vi "ABB Efficiency.vi"(11 "auto save":bool) -> ()   [LabVIEW 2017]
uses:
  <vilib>/Analysis/baseanly.llb/Mean (DBL).vi
  ABB global.vi
  <vilib>/Analysis/NI_AALBase.lvlib
panel:
  in  "Slip Entry":dbl[](array[numeric])=[0.0, 0.0, 0.0, 0.0]
  in  "Slip Source":enum16{"Calculated", "Entered"}(ring)
  in  "Specified dTs":cluster{" Stator":string, "Rotor":string}
  in  "Calculated Temperature Rise":cluster{" Stator dT":dbl, "Rotor dT":dbl}
  out "Ambient temp":dbl
  in  "Specified Efficiencies (%)":dbl[](array[numeric])=[0.0, 0.0, 0.0, 0.0]
  in  "Specified  Power Factor":dbl[](array[numeric])=[0.0, 0.0, 0.0, 0.0]
  in  "Temperature Rise Settings":T1
  in  "Frequency (Hz)":dbl
  in  "Remarks":string
  out "Pass/Fail Criteria":string[][](table)
  out "Efficiency Standard":u16(ring) items=["IEC 60034", "NEMA", "IEC 61972"]
  out "Selected Loads (% Rated)":dbl[](array[numeric])
  out "Loads (% Rated)":dbl[](array[numeric])
  out "Efficiency Readings":dbl[][](array[numeric]) format="%#.4f"
  in  "Load selection":bool[](array[boolean])=[FALSE, FALSE, FALSE, FALSE, FALSE]
  out "Stator Resistance/phase":dbl format="%#.6f"
  out "Losses at rated voltage":T2 {"Iron loss" format="%#.2f"; "No-Load Current" format="%#.2f"; "Total No load Power" format="%#.2f"; "Mech Loss" format="%#.3f"}
  out "Rated Data":T3 {"Slip" format="%#.5f"}
  in  "Exit":bool
  # "Efficiency Calculations & Pass/Fail Criteria"
  # "Efficiency"
  # "@"
  # "Calculated slip"
  # "Mechanical Loss  (kW)"
  # "Iron Loss (kW)"
  # "Stator Copper Loss (kW)"
  # "Rotor Copper Loss (kW)"
  # "Stray load loss (kW)"
  # "Total loss (kW)"
  # "Load (kW)"
  # "Efficiency (%)"
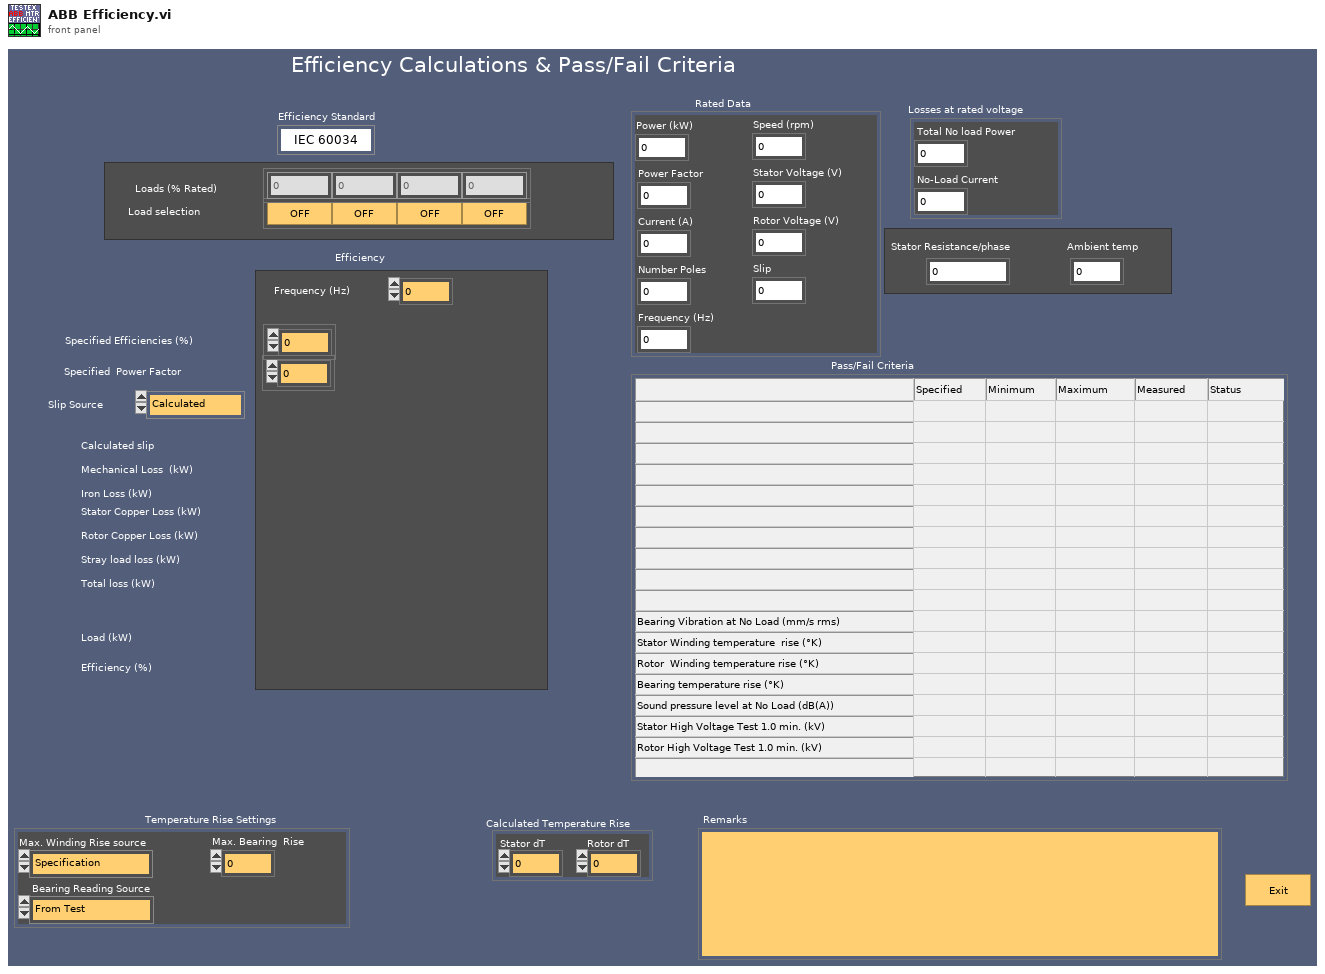
[diagram p1: front panel]
types:
  T1 = cluster{"Max. Winding Rise source":enum16{"Specification", "Enter"}, "Max.Winding Rise":dbl, " Max. Bearing  Rise":dbl, "Bearing Reading Source":enum16{"From Test", "Enter"}, "Bearing reading":dbl}
  T2 = cluster{"Mech Loss":dbl, "Total No load Power":dbl, "No-Load Current":dbl, "Iron loss":dbl}
  T3 = cluster{"Power (kW)":dbl, "Speed (rpm)":dbl, "Power Factor":dbl, "Stator Voltage (V)":dbl, "Current (A)":dbl, "Frequency (Hz)":dbl, "Number Poles":dbl, "Slip":dbl, "Rotor Voltage (V)":dbl}
  T4 = cluster{"Integer":i32, "Dbl":dbl, "String":string, "Boolean":bool}
  T5 = cluster{"Number of Loads":i32, "Loads (%Rated)":dbl[]}
  T6 = cluster{"PCu":dbl, "Pmech":dbl, "PFe":dbl, "Ptot":dbl, "Ambient":dbl, "I1":dbl, "I2":dbl, "I3":dbl, "Wdg Temp":dbl}
  T7 = cluster{"Slip Source":enum16{"Calculated", "Entered"}, "Slip Entry":dbl[]}
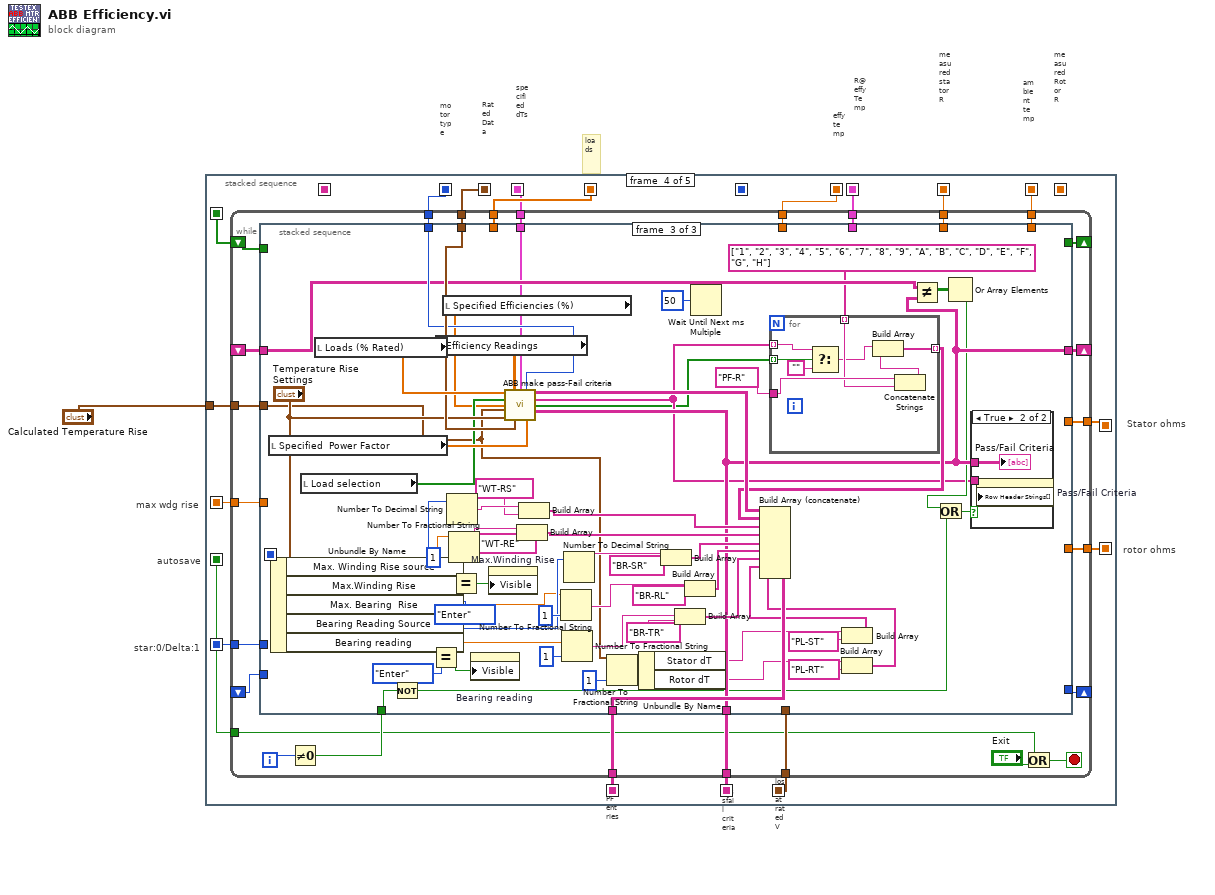
[diagram p0: block diagram]
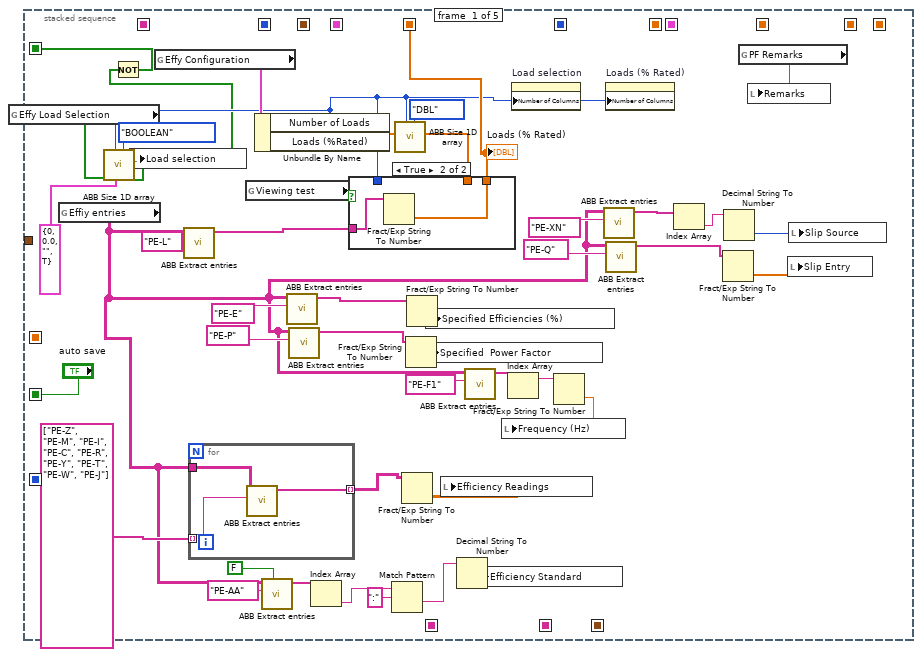
[diagram p2: hidden frame]
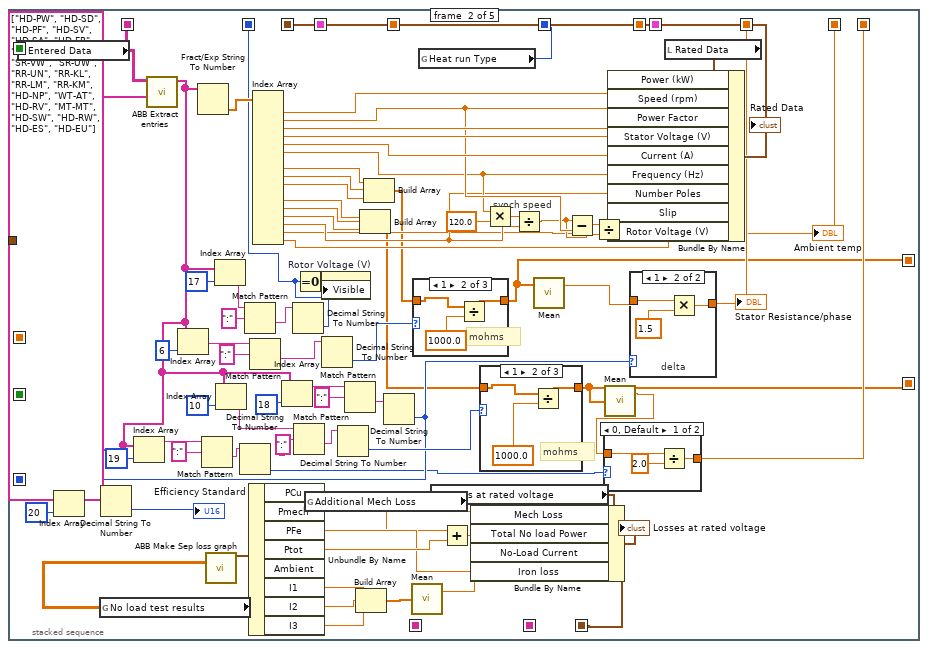
[diagram p4: hidden frame]
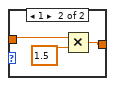
[diagram p5: hidden frame]
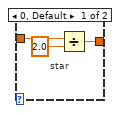
[diagram p6: hidden frame]
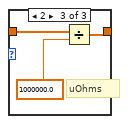
[diagram p8: hidden frame]
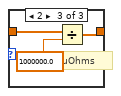
[diagram p10: hidden frame]
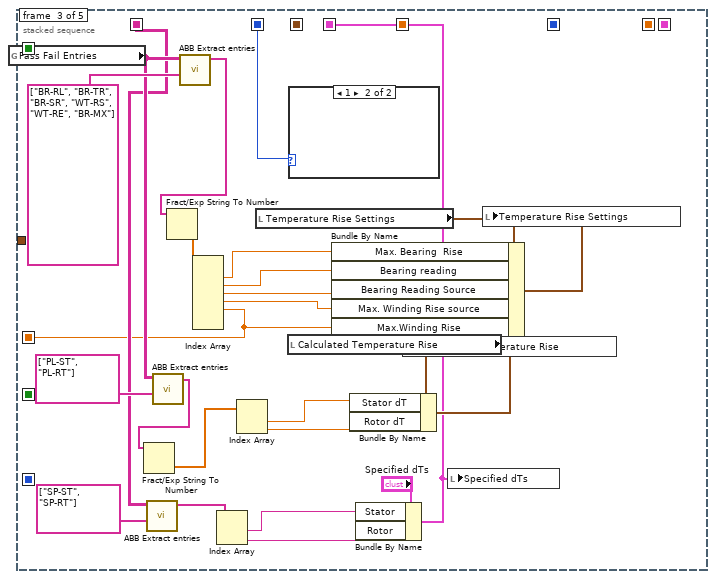
[diagram p11: hidden frame]
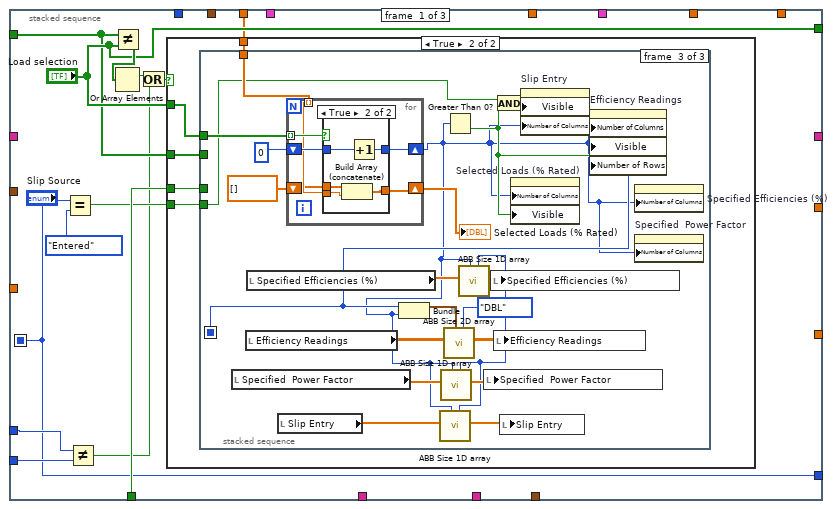
[diagram p13: hidden frame]
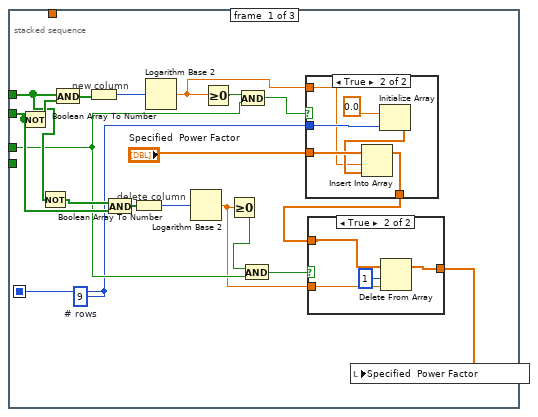
[diagram p15: hidden frame]
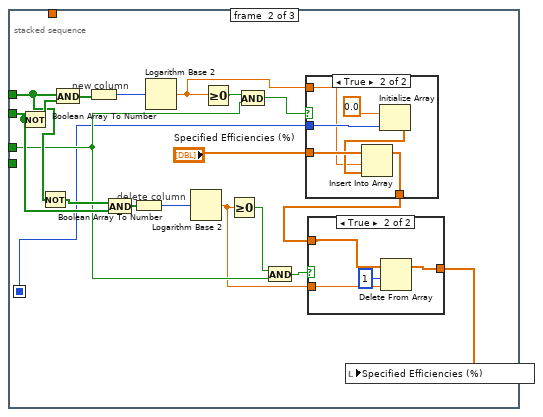
[diagram p18: hidden frame]
diagram:
  # "max wdg rise"
  # "specified dTs"
  # "R@ effy Temp"
  # "rotor ohms"
  # "Stator ohms"
  # "effy temp"
  # "measured Rotor R"
  # "ambient temp"
  # "star:0/Delta:1"
  # "measured stator R"
  # "motor type"
  # "autosave"
  # "PF entries"
  # "passfail criteria"
  # "Rated Data"
  # "losses at rated V"
  # "loads"
  n1 = stacked-sequence {
    seq-local: [w42 _ _ _ _] -> [_ _ _ w199 _]
    seq-local: [w37 _ _ _ _] -> [_ _ _ w198 _]
    seq-local: [_ w110 _ _ _] -> [_ _ _ w197 w432]
    seq-local: [_ w100 _ _ _] -> [_ _ _ w196 _]
    seq-local: [_ _ _ w195 _] -> [_ _ _ _ w438]
    seq-local: [_ _ _ w194 _] -> [_ _ _ _ w437]
    seq-local: [_ w91 _ _ _] -> [_ _ _ _ _]
    seq-local: ["auto save" _ _ _ _] -> [_ _ _ w193 w434]
    seq-local: [_ w81 _ _ _] -> [_ _ w181 w192 _]
    seq-local: [_ w80 _ _ _] -> [_ _ w163 _ _]
    seq-local: [_ w74 _ _ _] -> [_ _ _ w191 _]
    seq-local: [_ w72 _ _ _] -> [_ _ _ w190 _]
    seq-local: [_ w71 _ _ _] -> [_ _ _ w189 _]
    seq-local: [_ w65 _ _ _] -> [_ _ _ _ _]
    seq-local: [_ _ _ w188 _] -> [_ _ _ _ w431]
    seq-local: [_ w60 _ _ _] -> [_ _ _ w186 _]
    seq-local: [_ w59 _ _ _] -> [_ _ _ w185 _]
    seq-local: [_ _ _ w187 _] -> [_ _ _ _ w430]
    seq-local: [_ _ w157 _ _] -> [_ _ _ w184 _]
    seq-local: [_ _ w156 _ _] -> [_ _ _ w183 _]
    tunnel: "Calculated Temperature Rise" -> [_ _ _ w182 _]
    frame #0 {
      n2 = global read "ABB global.vi" "Effy Load Selection"() -> (w14:bool[])
      n3 = global read "ABB global.vi" "Effiy entries"() -> (w4:string[][])
      n4 = global read "ABB global.vi" "Effy Configuration"() -> (w45:T5)
      n5 = call "ABB Extract entries.vi"("Entry ID"="PE-L", "Entry table in"=w4) -> ("Selected Entries"=w39:string[])  [unwired: 9 in]
      n6 = for {
        tunnel: w4 -> [w48]
        tunnel: string[] ["PE-Z", "PE-M", "PE-I", "PE-C", "PE-R", "PE-Y", "PE-T", "PE-W", "PE-J"] -> [w47] mode=indexing
        tunnel: [w46] -> w34 mode=indexing
        n7 = call "ABB Extract entries.vi"("Entry ID"=w47, "Entry table in"=w48) -> ("Selected Entries"=w46:string[])  [unwired: 9 in]
      }
      n8 = global read "ABB global.vi" "Viewing test"() -> (w40:bool)
      n9 = Unbundle By Name(w45) -> ("Number of Loads"=w11:i32, "Loads (%Rated)"=w44:dbl[])
      n10 = call "ABB Size 1D array.vi"("Type"=enum16{"Integer", "DBL", "STRING", "BOOLEAN"}."BOOLEAN", "Default"=T4 {"Integer"=0, "Dbl"=0.0, "String"="", "Boolean"=TRUE}, "Size"=w11, "Boolean Array in"=w14) -> ("Boolean Array out"=w10:bool[])  [unwired: 4 in, 3 out]
      n11 = Not(x=w10) -> (.not. x?=w42:bool[])
      n12 = local write "Load selection"(w10) -> ()
      n13 = call "ABB Extract entries.vi"("Pulldown text"=FALSE, "Entry ID"="PE-AA", "Entry table in"=w4) -> ("Selected Entries"=w30:string[])  [unwired: 8 in]
      n14 = call "ABB Extract entries.vi"("Entry ID"="PE-E", "Entry table in"=w4) -> ("Selected Entries"=w33:string[])  [unwired: 9 in]
      n15 = call "ABB Extract entries.vi"("Entry ID"="PE-P", "Entry table in"=w4) -> ("Selected Entries"=w17:string[])  [unwired: 9 in]
      n16 = Index Array(array=w30) -> (element=w29:string)  [unwired: 1 in]
      n17 = Match Pattern(string=w29, regular expression=":") -> (after substring=w19:string)  [unwired: 1 in, 3 out]
      n18 = call "ABB Size 1D array.vi"("Type"=enum16{"Integer", "DBL", "STRING", "BOOLEAN"}."DBL", "Size"=w11, "DBL Array In"=w44) -> ("DBL Array out"=w38:dbl[])  [unwired: 5 in, 3 out]
      n19 = case shown="True" w40 {
        tunnel: w39 -> [_ w51]
        tunnel: w38 -> [w49 _]
        tunnel: [w49 w50] -> w37
        tunnel: w11 -> [_ _]
        frame False {
        }
        frame True {
          n20 = Fract/Exp String To Number(string=w51) -> (number=w50:dbl[])  [unwired: 3 in, 1 out]
        }
      }
      "Loads (% Rated)" <- w37
      n21 = Fract/Exp String To Number(string=w34) -> (number=w35:dbl[][])  [unwired: 3 in, 1 out]
      n22 = Fract/Exp String To Number(string=w17) -> (number=w16:dbl[])  [unwired: 3 in, 1 out]
      n23 = Fract/Exp String To Number(string=w33) -> (number=w15:dbl[])  [unwired: 3 in, 1 out]
      n24 = local write "Specified  Power Factor"(w16) -> ()
      n25 = local write "Specified Efficiencies (%)"(w15) -> ()
      n26 = local write "Efficiency Readings"(w35) -> ()
      n27 = Decimal String To Number(string=w19) -> (number=w27:i32)  [unwired: 2 in, 1 out]
      n28 = call "ABB Extract entries.vi"("Entry ID"="PE-F1", "Entry table in"=w4) -> ("Selected Entries"=w23:string[])  [unwired: 9 in]
      n29 = local write "Efficiency Standard"(w27) -> ()
      n30 = Index Array(array=w23) -> (element=w22:string)  [unwired: 1 in]
      n31 = property on="Load selection" class="Arr (strict)"("Number of Columns"=w11) -> ()  [unwired: 2 in, 2 out]
      n32 = Fract/Exp String To Number(string=w22) -> (number=w21:dbl)  [unwired: 3 in, 1 out]
      n33 = local write "Frequency (Hz)"(w21) -> ()
      n34 = call "ABB Extract entries.vi"("Entry ID"="PE-XN", "Entry table in"=w4) -> ("Selected Entries"=w5:string[])  [unwired: 9 in]
      n35 = property on="Loads (% Rated)" class="Arr (strict)"("Number of Columns"=w11) -> ()  [unwired: 2 in, 2 out]
      n36 = call "ABB Extract entries.vi"("Entry ID"="PE-Q", "Entry table in"=w4) -> ("Selected Entries"=w8:string[])  [unwired: 9 in]
      n37 = Index Array(array=w5) -> (element=w3:string)  [unwired: 1 in]
      n38 = Fract/Exp String To Number(string=w8) -> (number=w9:dbl[])  [unwired: 3 in, 1 out]
      n39 = Decimal String To Number(string=w3) -> (number=w2:i32)  [unwired: 2 in, 1 out]
      n40 = global read "ABB global.vi" "PF Remarks"() -> (w20:string)
      n41 = local write "Remarks"(w20) -> ()
      n42 = local write "Slip Entry"(w9) -> ()
      n43 = local write "Slip Source"(w2) -> ()
    }
    frame #1 {
      # "synch speed"
      n44 = global read "ABB global.vi" "Entered Data"() -> (w80:string[][])
      n45 = global read "ABB global.vi" "No load test results"() -> (w90:dbl[][])
      n46 = call "ABB Extract entries.vi"("Entry IDs"=string[] ["HD-PW", "HD-SD", "HD-PF", "HD-SV", "HD-SA", "HD-FR", "SR-UN", "SR-UV", "SR-VW", "SR-UW", "RR-UN", "RR-KL", "RR-LM", "RR-KM", "HD-NP", "WT-AT", "HD-RV", "MT-MT", "HD-SW", "HD-RW", "HD-ES", "HD-EU"] ("Array"), "Entry table in"=w80) -> ("Selected Entries"=w57:string[])  [unwired: 9 in]
      n47 = Index Array(array=w57, index=20) -> (element=w56:string)
      n48 = Decimal String To Number(string=w56) -> (number=→"Efficiency Standard":i32)  [unwired: 2 in, 1 out]
      n49 = Index Array(array=w57, index=19) -> (element=w70:string)
      n50 = Index Array(array=w57, index=6) -> (element=w112:string)
      n51 = Fract/Exp String To Number(string=w57) -> (number=w114:dbl[])  [unwired: 3 in, 1 out]
      n52 = Match Pattern(string=w70, regular expression=":") -> (after substring=w66:string)  [unwired: 1 in, 3 out]
      n53 = call "ABB Make Sep loss graph.vi"("Results"=w90) -> ("Rated V Readings"=w124:T6)  [unwired: 8 in, 2 out]
      n54 = Index Array(array=w57, index=17) -> (element=w86:string)
      n55 = Index Array(array=w57, index=10) -> (element=w106:string)
      n56 = Decimal String To Number(string=w66) -> (number=w67:i32)  [unwired: 2 in, 1 out]
      n57 = Match Pattern(string=w86, regular expression=":") -> (after substring=w84:string)  [unwired: 1 in, 3 out]
      n58 = Unbundle By Name(w124) -> ("Pmech"=w52:dbl, "PFe"=w108:dbl, "Ptot"=w123:dbl, "I1"=w122:dbl, "I2"=w121:dbl, "I3"=w120:dbl)  [unwired: 2 out]
      n59 = Match Pattern(string=w112, regular expression=":") -> (after substring=w83:string)  [unwired: 1 in, 3 out]
      n60 = Index Array(array=w114) -> (element #1=w128:dbl, element #2=w99:dbl, element #3=w127:dbl, element #4=w126:dbl, element #5=w125:dbl, element #6=w96:dbl, element #8=w117:dbl, element #9=w116:dbl, element #10=w115:dbl, element #12=w103:dbl, element #13=w102:dbl, element #14=w101:dbl, element #15=w93:dbl, element #16=w71:dbl, element #17=w89:dbl)  [unwired: 17 in, 2 out]
      "Ambient temp" <- w71
      n61 = Index Array(array=w57, index=18) -> (element=w76:string)
      n62 = Decimal String To Number(string=w84) -> (number=w81:i32)  [unwired: 2 in, 1 out]
      n63 = Match Pattern(string=w106, regular expression=":") -> (after substring=w82:string)  [unwired: 1 in, 3 out]
      n64 = Equal To 0?(x=w81) -> (x = 0?=w88:bool)
      n65 = global read "ABB global.vi" "Additional Mech Loss"() -> (w53:dbl)
      n66 = property on="Rotor Voltage (V)" class="DigNum (strict)"("Visible"=w88) -> ()  [unwired: 2 in, 2 out]
      n67 = Decimal String To Number(string=w83) -> (number=w73:i32)  [unwired: 2 in, 1 out]
      n68 = Decimal String To Number(string=w82) -> (number=w104:i32)  [unwired: 2 in, 1 out]
      n69 = Match Pattern(string=w76, regular expression=":") -> (after substring=w78:string)  [unwired: 1 in, 3 out]
      n70 = Build Array(w122, w121, w120) -> (w119:dbl[])
      n71 = Build Array(w103, w102, w101) -> (w62:dbl[])
      n72 = Build Array(w117, w116, w115) -> (w64:dbl[])
      n73 = Decimal String To Number(string=w78) -> (number=w72:i32)  [unwired: 2 in, 1 out]
      n74 = call-poly <vilib>:"Mean.vi"("X"=w119) -> ("mean"=w75:dbl)  [unwired: 1 out]
      n75 = case shown="1" w73 {
        tunnel: w64 -> [w149 w152 w155]
        tunnel: [w149 w150 w153] -> w60
        frame 0, Default {
          # "ohms"
        }
        frame 1 {
          # "mohms"
          n76 = Divide(x=w152, y=1000.0) -> (x/y=w150:dbl[])
        }
        frame 2 {
          # "uOhms"
          n77 = Divide(x=w155, y=1000000.0) -> (x/y=w153:dbl[])
        }
      }
      n78 = global read "ABB global.vi" "Heat run Type"() -> (w91:enum16{"Full Load", "Partial- & No-Load"})
      n79 = local read "Losses at rated voltage"() -> (w129:T2)
      n80 = Add(x=w53, y=w123) -> (x+y=w54:dbl)
      n81 = Bundle By Name(cluster=w129, "Mech Loss"=w52, "Total No load Power"=w54, "No-Load Current"=w75, "Iron loss"=w108) -> (w110:T2)
      "Losses at rated voltage" <- w110
      n82 = case shown="1" w104 {
        tunnel: w62 -> [w142 w145 w148]
        tunnel: [w142 w143 w146] -> w59
        frame 0, Default {
          # "ohms"
        }
        frame 1 {
          # "mohms"
          n83 = Divide(x=w145, y=1000.0) -> (x/y=w143:dbl[])
        }
        frame 2 {
          # "uOhms"
          n84 = Divide(x=w148, y=1000000.0) -> (x/y=w146:dbl[])
        }
      }
      n85 = Multiply(x=w96, y=120.0) -> (x*y=w94:dbl)
      n86 = Divide(x=w94, y=w93) -> (x/y=w92:dbl)
      n87 = call-poly <vilib>:"Mean.vi"("X"=w60) -> ("mean"=w63:dbl)  [unwired: 1 out]
      n88 = Subtract(x=w92, y=w99) -> (x-y=w98:dbl)
      n89 = Divide(x=w98, y=w92) -> (x/y=w97:dbl)
      n90 = call-poly <vilib>:"Mean.vi"("X"=w59) -> ("mean"=w61:dbl)  [unwired: 1 out]
      n91 = case shown="0, Default" w67 {
        tunnel: w61 -> [w131 w133]
        tunnel: [w130 w135] -> w65
        frame 0, Default {
          n92 = Divide(x=w131, y=2.0) -> (x/y=w130:dbl)
        }
        frame 1 {
          n93 = Multiply(x=w133, y=1.5) -> (x*y=w135:dbl)
        }
      }
      n94 = case shown="1" w72 {
        tunnel: w63 -> [w138 w141]
        tunnel: [w136 w140] -> w74
        frame 0, Default {
          # "star"
          n95 = Divide(x=w138, y=2.0) -> (x/y=w136:dbl)
        }
        frame 1 {
          # "delta"
          n96 = Multiply(x=w141, y=1.5) -> (x*y=w140:dbl)
        }
      }
      "Stator Resistance/phase" <- w74
      n97 = local read "Rated Data"() -> (w109:T3)
      n98 = Bundle By Name(cluster=w109, "Power (kW)"=w128, "Speed (rpm)"=w99, "Power Factor"=w127, "Stator Voltage (V)"=w126, "Current (A)"=w125, "Frequency (Hz)"=w96, "Number Poles"=w93, "Slip"=w97, "Rotor Voltage (V)"=w89) -> (w100:T3)
      "Rated Data" <- w100
    }
    frame #2 {
      n99 = global read "ABB global.vi" "Pass Fail Entries"() -> (w169:string[][])
      n100 = call "ABB Extract entries.vi"("Entry IDs"=string[] ["SP-ST", "SP-RT"], "Entry table in"=w163) -> ("Selected Entries"=w161:string[])  [unwired: 9 in]
      n101 = call "ABB Extract entries.vi"("Entry IDs"=string[] ["PL-ST", "PL-RT"], "Entry table in"=w169) -> ("Selected Entries"=w168:string[])  [unwired: 9 in]
      n102 = Fract/Exp String To Number(string=w168) -> (number=w166:dbl[])  [unwired: 3 in, 1 out]
      n103 = call "ABB Extract entries.vi"("Entry IDs"=string[] ["BR-RL", "BR-TR", "BR-SR", "WT-RS", "WT-RE", "BR-MX"], "Entry table in"=w169) -> ("Selected Entries"=w179:string[])  [unwired: 9 in]
      n104 = Fract/Exp String To Number(string=w179) -> (number=w178:dbl[])  [unwired: 3 in, 1 out]
      n105 = Index Array(array=w178) -> (element #1=w175:dbl, element #2=w173:dbl, element #3=w172:dbl, element #4=w174:dbl, element #5=w156:dbl)  [unwired: 7 in, 2 out]
      n106 = Index Array(array=w161) -> (element #1=w159:string, element #2=w158:string)  [unwired: 2 in]
      n107 = Index Array(array=w166) -> (element #1=w165:dbl, element #2=w164:dbl)  [unwired: 2 in]
      n108 = local read "Temperature Rise Settings"() -> (w177:T1)
      n109 = local read "Calculated Temperature Rise"() -> (w171:cluster{" Stator dT":dbl, "Rotor dT":dbl})
      n110 = case shown="1" w181 {
        frame 0, Default {
        }
        frame 1 {
        }
      }
      n111 = Bundle By Name(cluster=w177, "Max. Bearing  Rise"=w175, "Bearing reading"=w173, "Bearing Reading Source"=w172, "Max. Winding Rise source"=w174, "Max.Winding Rise"=w156) -> (w176:T1)
      n112 = Bundle By Name(cluster=w171, "Stator dT"=w165, "Rotor dT"=w164) -> (w170:cluster{" Stator dT":dbl, "Rotor dT":dbl})
      n113 = Bundle By Name(cluster="Specified dTs", "Stator"=w159, "Rotor"=w158) -> (w157:cluster{" Stator":string, "Rotor":string})
      n114 = local write "Calculated Temperature Rise"(w170) -> ()
      n115 = local write "Specified dTs"(w157) -> ()
      n116 = local write "Temperature Rise Settings"(w176) -> ()
    }
    frame #3 {
      n117 = while {
        shift-right: [w224] -> _
        shift-left: w199 -> [w225]
        tunnel: w198 -> [w223]
        tunnel: w197 -> [w220]
        tunnel: w196 -> [w219]
        tunnel: [w218] -> w195
        tunnel: [w217] -> w194
        tunnel: w193 -> [w215]
        tunnel: w192 -> [w214]
        tunnel: w191 -> [w213]
        shift-right: [w211] -> _
        shift-left: _ -> [w212]
        tunnel: w190 -> [w210]
        tunnel: w189 -> [w209]
        tunnel: [w208] -> w188
        tunnel: [w207] -> w187
        tunnel: w186 -> [w206]
        tunnel: w185 -> [w205]
        tunnel: w184 -> [w204]
        shift-right: [w203] -> _
        shift-left: _ -> [w202]
        tunnel: w183 -> [w201]
        tunnel: w182 -> [w200]
        i -> [w222]
        stop <- w216 stop-if-true
        n118 = Not Equal To 0?(x=w222) -> (x != 0?=w221:bool)
        n119 = stacked-sequence {
          seq-local: ["Slip Source" _ _] -> [_ w344 _]
          tunnel: w225 -> [w236 _ _]
          tunnel: ["Load selection" _ _] -> w224
          tunnel: w223 -> [w237 _ _]
          tunnel: w221 -> [w235 _ w379]
          tunnel: w220 -> [_ w356 _]
          tunnel: w219 -> [_ w357 w417]
          tunnel: [_ _ w381] -> w218
          tunnel: [_ _ w412] -> w217
          tunnel: w214 -> [_ _ w414]
          tunnel: w213 -> [_ w355 _]
          tunnel: w212 -> [_ _ w382]
          tunnel: [_ _ w381] -> w211
          tunnel: w210 -> [w231 w352 _]
          tunnel: w209 -> [_ w351 _]
          tunnel: [_ w350 _] -> w208
          tunnel: [_ w349 _] -> w207
          tunnel: w206 -> [_ w348 _]
          tunnel: w205 -> [_ w347 _]
          tunnel: w204 -> [_ _ w361]
          tunnel: ["Slip Source" _ _] -> w203
          tunnel: w202 -> [w232 _ _]
          tunnel: w201 -> [_ _ _]
          tunnel: w200 -> [_ w341 w360]
          frame #0 {
            n120 = Equal?(x="Slip Source", y=enum16{"Calculated", "Entered"}."Entered") -> (x = y?=w233:bool)
            n121 = Not Equal?(x=w231, y=w232) -> (x != y?=w228:bool)
            n122 = Not Equal?(x=w236, y="Load selection") -> (x != y?=w239:bool[])
            n123 = Or Array Elements(Boolean array=w239) -> (logical OR=w229:bool)
            n124 = Or(x=w229, y=w228) -> (x .or. y?=w230:bool)
            n125 = case shown="True" w230 {
              tunnel: "Load selection" -> [_ w243]
              tunnel: w237 -> [_ w244]
              tunnel: w236 -> [_ w242]
              tunnel: w235 -> [_ w241]
              tunnel: w233 -> [_ w240]
              frame False {
              }
              frame True {
                n126 = stacked-sequence {
                  seq-local: [w245 _ _] -> [_ w277 w318]
                  tunnel: w244 -> [_ _ w326]
                  tunnel: w243 -> [w257 w288 w325]
                  tunnel: w242 -> [w255 w286 _]
                  tunnel: w241 -> [w250 w281 _]
                  tunnel: w240 -> [_ _ w311]
                  frame #0 {
                    w245 = 9  # # rows
                    # "delete column"
                    # "new column"
                    n127 = Not(x=w255) -> (.not. x?=w263:bool[])
                    n128 = Not(x=w257) -> (.not. x?=w256:bool[])
                    n129 = And(x=w257, y=w263) -> (x .and. y?=w262:bool[])
                    n130 = Boolean Array To Number(Boolean array=w262) -> (number=w261:u32)
                    n131 = And(x=w256, y=w255) -> (x .and. y?=w253:bool[])
                    n132 = Boolean Array To Number(Boolean array=w253) -> (number=w254:u32)
                    n133 = Logarithm Base 2(1:w261) -> (0:w258:dbl)
                    n134 = Logarithm Base 2(1:w254) -> (0:w248:dbl)
                    n135 = Greater Or Equal To 0?(x=w258) -> (x >= 0?=w260:bool)
                    n136 = Greater Or Equal To 0?(x=w248) -> (x >= 0?=w249:bool)
                    n137 = And(x=w260, y=w250) -> (x .and. y?=w259:bool)
                    n138 = And(x=w249, y=w250) -> (x .and. y?=w251:bool)
                    n139 = case shown="True" w259 {
                      tunnel: "Specified  Power Factor" -> [w269 w275]
                      tunnel: w258 -> [_ w270]
                      tunnel: w245 -> [_ w273]
                      tunnel: [w269 w272] -> w252
                      frame False {
                      }
                      frame True {
                        n140 = Initialize Array(0.0, w273) -> (w271:dbl[])
                        n141 = Insert Into Array(array=w275, index=w270, new element=w271) -> (w272:dbl[])
                      }
                    }
                    n142 = case shown="True" w251 {
                      tunnel: w252 -> [w264 w268]
                      tunnel: w248 -> [_ w265]
                      tunnel: [w264 w267] -> w247
                      frame False {
                      }
                      frame True {
                        n143 = Delete From Array(array=w268, length=1, index=w265) -> (array with subset deleted=w267:dbl[])  [unwired: 1 out]
                      }
                    }
                    n144 = local write "Specified  Power Factor"(w247) -> ()
                  }
                  frame #1 {
                    # "delete column"
                    # "new column"
                    n145 = Not(x=w286) -> (.not. x?=w294:bool[])
                    n146 = Not(x=w288) -> (.not. x?=w287:bool[])
                    n147 = And(x=w288, y=w294) -> (x .and. y?=w293:bool[])
                    n148 = Boolean Array To Number(Boolean array=w293) -> (number=w292:u32)
                    n149 = And(x=w287, y=w286) -> (x .and. y?=w284:bool[])
                    n150 = Boolean Array To Number(Boolean array=w284) -> (number=w285:u32)
                    n151 = Logarithm Base 2(1:w292) -> (0:w289:dbl)
                    n152 = Logarithm Base 2(1:w285) -> (0:w279:dbl)
                    n153 = Greater Or Equal To 0?(x=w289) -> (x >= 0?=w291:bool)
                    n154 = Greater Or Equal To 0?(x=w279) -> (x >= 0?=w280:bool)
                    n155 = And(x=w291, y=w281) -> (x .and. y?=w290:bool)
                    n156 = And(x=w280, y=w281) -> (x .and. y?=w282:bool)
                    n157 = case shown="True" w290 {
                      tunnel: "Specified Efficiencies (%)" -> [w300 w306]
                      tunnel: w289 -> [_ w301]
                      tunnel: w277 -> [_ w304]
                      tunnel: [w300 w303] -> w283
                      frame False {
                      }
                      frame True {
                        n158 = Initialize Array(0.0, w304) -> (w302:dbl[])
                        n159 = Insert Into Array(array=w306, index=w301, new element=w302) -> (w303:dbl[])
                      }
                    }
                    n160 = case shown="True" w282 {
                      tunnel: w283 -> [w295 w299]
                      tunnel: w279 -> [_ w296]
                      tunnel: [w295 w298] -> w278
                      frame False {
                      }
                      frame True {
                        n161 = Delete From Array(array=w299, length=1, index=w296) -> (array with subset deleted=w298:dbl[])  [unwired: 1 out]
                      }
                    }
                    n162 = local write "Specified Efficiencies (%)"(w278) -> ()
                  }
                  frame #2 {
                    w308 = enum16{"Integer", "DBL", "STRING", "BOOLEAN"}."DBL" ("Type")
                    n163 = local read "Specified  Power Factor"() -> (w316:dbl[])
                    n164 = local read "Efficiency Readings"() -> (w319:dbl[][])
                    n165 = local read "Specified Efficiencies (%)"() -> (w315:dbl[])
                    n166 = local read "Slip Entry"() -> (w310:dbl[])
                    n167 = for {
                      tunnel: w326 -> [w329] mode=indexing
                      tunnel: w325 -> [w332] mode=indexing
                      shift-right: [w330] -> w309
                      shift-left: 0 -> [w331]
                      shift-right: [w328] -> w322
                      shift-left: dbl[] [] -> [w327]
                      n168 = case shown="True" w332 {
                        tunnel: w331 -> [w334 w339]
                        tunnel: [w334 w338] -> w330
                        tunnel: w329 -> [_ w336]
                        tunnel: [w333 w335] -> w328
                        tunnel: w327 -> [w333 w337]
                        frame False {
                        }
                        frame True {
                          n169 = Build Array (concatenate)(w337, w336) -> (w335:dbl[])
                          n170 = Increment(x=w339) -> (x+1=w338:i32)
                        }
                      }
                    }
                    "Selected Loads (% Rated)" <- w322
                    n171 = Bundle("# rows"=w318, w309) -> (w321:cluster{"# rows":i32, i32})  [unwired: 1 in]
                    n172 = call "ABB Size 1D array.vi"("Type"=w308, "Size"=w309, "DBL Array In"=w310) -> ("DBL Array out"=w307:dbl[])  [unwired: 5 in, 3 out]
                    n173 = call "ABB Size 1D array.vi"("Type"=w308, "Size"=w309, "DBL Array In"=w316) -> ("DBL Array out"=w317:dbl[])  [unwired: 5 in, 3 out]
                    n174 = call "ABB Size 2D array.vi"("Type"=w308, "Size"=w321, "DBL Array In"=w319) -> ("DBL Array out"=w320:dbl[][])  [unwired: 5 in, 3 out]
                    n175 = Greater Than 0?(x=w309) -> (x > 0?=w313:bool)
                    n176 = call "ABB Size 1D array.vi"("Type"=w308, "Size"=w309, "DBL Array In"=w315) -> ("DBL Array out"=w314:dbl[])  [unwired: 5 in, 3 out]
                    n177 = local write "Specified  Power Factor"(w317) -> ()
                    n178 = local write "Specified Efficiencies (%)"(w314) -> ()
                    n179 = And(x=w311, y=w313) -> (x .and. y?=w312:bool)
                    n180 = local write "Efficiency Readings"(w320) -> ()
                    n181 = local write "Slip Entry"(w307) -> ()
                    n182 = property on="Selected Loads (% Rated)" class="Arr (strict)"("Number of Columns"=w309, "Visible"=w313) -> ()  [unwired: 2 in, 2 out]
                    n183 = property on="Slip Entry" class="Arr (strict)"("Visible"=w312, "Number of Columns"=w309) -> ()  [unwired: 2 in, 2 out]
                    n184 = property on="Efficiency Readings" class="Arr (strict)"("Number of Columns"=w309, "Visible"=w313, "Number of Rows"=w318) -> ()  [unwired: 2 in, 2 out]
                    n185 = property on="Specified Efficiencies (%)" class="Arr (strict)"("Number of Columns"=w309) -> ()  [unwired: 2 in, 2 out]
                    n186 = property on="Specified  Power Factor" class="Arr (strict)"("Number of Columns"=w309) -> ()  [unwired: 2 in, 2 out]
                  }
                }
              }
            }
          }
          frame #1 {
            n187 = Unbundle By Name(w341) -> ("Stator dT"=w340:dbl)
            n188 = local read "Selected Loads (% Rated)"() -> (w358:dbl[])
            n189 = local read "Specified  Power Factor"() -> (w359:dbl[])
            n190 = local read "Efficiency Standard"() -> (w342:u16)
            n191 = local read "Frequency (Hz)"() -> (w354:dbl)
            n192 = Bundle("Slip Source"=w344, "Slip Entry"="Slip Entry") -> (w343:T7)  [unwired: 1 in]
            n193 = Bundle(w348, w347) -> (w346:cluster{dbl[], dbl[]})  [unwired: 1 in]
            n194 = call "ABB Calc efficiency2.vi"("Rated Data"=w357, "max wdg rise"=w340, "Stator wdg"=w352, "Stator  Phase resistance"=w355, "Ambient temp"=w351, "Frequency (Hz)"=w354, "Efficiency Standard"=w342, "Specified  Power Factor"=w359, "Selected Loads (% Rated)"=w358, "Ohms"=w346, "Losses at rated voltage"=w356, "slip entry"=w343) -> ("Efficiency out"=→"Efficiency Readings":dbl[][], "Effy Temp"=w350:dbl, "R at EffyT"=w349:cluster{"Stator":dbl[], "Rotor":dbl[]})  [unwired: 1 in]
          }
          frame #2 {
            n195 = local read "Specified  Power Factor"() -> (w374:dbl[])
            n196 = Unbundle By Name("Temperature Rise Settings") -> ("Max. Winding Rise source"=w406:enum16{"Specification", "Enter"}, "Max.Winding Rise"=w405:dbl, "Max. Bearing  Rise"=w385:dbl, "Bearing Reading Source"=w386:enum16{"From Test", "Enter"}, "Bearing reading"=w384:dbl)
            n197 = local read "Load selection"() -> (w373:bool[])
            n198 = local read "Loads (% Rated)"() -> (w419:dbl[])
            n199 = Not(x=w379) -> (.not. x?=w376:bool)
            n200 = Equal?(x=w386, y=enum16{"From Test", "Enter"}."Enter") -> (x = y?=w407:bool)
            n201 = local read "Efficiency Readings"() -> (w418:dbl[][])
            n202 = local read "Specified Efficiencies (%)"() -> (w371:dbl[])
            n203 = Number To Decimal String(number=w406) -> (decimal integer string=w403:string)  [unwired: 1 in]
            n204 = Number To Fractional String(number=w405, precision (6)=i16 1) -> (F-format string=w402:string)  [unwired: 2 in]
            n205 = Equal?(x=w406, y=enum16{"Specification", "Enter"}."Enter") -> (x = y?=w409:bool)
            n206 = property on="Bearing reading" class="DigNum (strict)"("Visible"=w407) -> ()  [unwired: 2 in, 2 out]
            n207 = property on="Max.Winding Rise" class="DigNum (strict)"("Visible"=w409) -> ()  [unwired: 2 in, 2 out]
            n208 = call "ABB make pass-Fail criteria.vi"("Loads (% Rated)"=w419, "Efficiency Readings"=w418, "spect temp rise"=w361, "motor type"=w414, "Load selection"=w373, "Specified Efficiencies (%)"=w371, "Partial load"=w360, "Temperature Rise Settings"="Temperature Rise Settings", "Rated Data"=w417, "Specified  Power Factor"=w374) -> ("Entries"=w416:string[][], "row headers"=w375:string[], "measurements taken"=w370:bool[], "Pass/Fail Criteria"=w381:string[][])  [unwired: 2 in]
            n209 = Build Array(w402, "WT-RE" ("element")) -> (w398:string[])
            n210 = Build Array(w403, "WT-RS") -> (w399:string[])
            n211 = Number To Fractional String(number=w385, precision (6)=i16 1) -> (F-format string=w394:string)  [unwired: 2 in]
            n212 = Number To Fractional String(number=w384, precision (6)=i16 1) -> (F-format string=w393:string)  [unwired: 2 in]
            n213 = Number To Decimal String(number=w386) -> (decimal integer string=w397:string)  [unwired: 1 in]
            n214 = Number To Fractional String(number=w360, precision (6)=i16 1) -> (F-format string=w369:cluster{" Stator dT":string, "Rotor dT":string})  [unwired: 2 in]
            n215 = Unbundle By Name(w369) -> ("Stator dT"=w366:string, "Rotor dT"=w365:string)
            n216 = Build Array(w397, "BR-SR") -> (w389:string[])
            n217 = Build Array(w393, "BR-TR" ("element")) -> (w387:string[])
            n218 = Build Array(w394, "BR-RL" ("element")) -> (w388:string[])
            n219 = Wait Until Next ms Multiple(millisecond multiple=u32 50) -> ()  [unwired: 1 out]
            n220 = for {
              tunnel: w375 -> [w424] mode=indexing
              tunnel: "PF-R" -> [w429]
              tunnel: [w427] -> w411 mode=indexing
              tunnel: string[] ["1", "2", "3", "4", "5", "6", "7", "8", "9", "A", "B", "C", "D", "E", "F", "G", "H"] -> [w426] mode=indexing
              tunnel: w370 -> [w425] mode=indexing
              n221 = Select(t=w424, s=w425, f="") -> (s? t:f=w422:string)
              n222 = Concatenate Strings(w429, w426) -> (w428:string)
              n223 = Build Array(w422, w428) -> (w427:string[])
            }
            n224 = Build Array(w366, "PL-ST" ("element")) -> (w363:string[])
            n225 = Build Array(w365, "PL-RT" ("element")) -> (w362:string[])
            n226 = Build Array (concatenate)(w416, w411, w399, w398, w389, w388, w387, w363, w362) -> (w412:string[][])
            n227 = Not Equal?(x=w382, y=w381) -> (x != y?=w380:bool[][])
            n228 = Or Array Elements(Boolean array=w380) -> (logical OR=w377:bool)
            n229 = Or(x=w377, y=w376) -> (x .or. y?=w378:bool)
            n230 = case shown="True" w378 {
              tunnel: w381 -> [_ w421]
              tunnel: w375 -> [_ w420]
              frame False {
              }
              frame True {
                n231 = property on="Pass/Fail Criteria" class="Tbl (strict)"("Row Header Strings[]"=w420) -> ()  [unwired: 2 in, 2 out]
                "Pass/Fail Criteria" <- w421
              }
            }
          }
        }
        n232 = Or(x=w215, y="Exit") -> (x .or. y?=w216:bool)
      }
    }
    frame #4 {
      # "No Load Readings\n 0 : I1\n 1 : I2\n 2 : I3\n 3 : Iav\n 4 : V1\n 5 : V2\n 6 : V3\n 7 : Vav\n 8 : Ptot\n 9 : Pf\n10 : Pcu\n11 : Pmech\n12 : Pfe\n13 : Pnold"
      n233 = global read "ABB global.vi" "Viewing test"() -> (w435:bool)
      n234 = Not(x=w434) -> (.not. x?=w433:bool)
      n235 = And(x=w435, y=w433) -> (x .and. y?=w436:bool)
      n236 = case shown="False" w436 {
        tunnel: w438 -> [w444 _]
        tunnel: w437 -> [w443 _]
        tunnel: w434 -> [w442 _]
        tunnel: w432 -> [w441 _]
        tunnel: w431 -> [w440 _]
        tunnel: w430 -> [w439 _]
        frame False {
          n237 = case shown="False" w442 {
            tunnel: [w449 TRUE ("T button?")] -> w446
            frame False {
              n238 = Two Button Dialog(message="Save results?", 1:"Discard" ("F button name (\"Cancel\")"), 2:"Save" ("T button name (\"OK\")")) -> (T button?=w449:bool)
            }
            frame True {
            }
          }
          n239 = global read "ABB global.vi" "Current test"() -> (w445:path)
          n240 = case shown="True" w446 {
            tunnel: w445 -> [_ w458]
            tunnel: w444 -> [_ w457]
            tunnel: w443 -> [_ w456]
            tunnel: w442 -> [_ w455]
            tunnel: w441 -> [_ w454]
            tunnel: w440 -> [_ w453]
            tunnel: w439 -> [_ w452]
            frame False {
            }
            frame True {
              n241 = stacked-sequence {
                seq-local: [w477 _ _ _ _] -> [_ w516 _ _ _]
                seq-local: [_ w510 _ _ _] -> [_ _ w563 _ _]
                seq-local: [_ _ w547 _ _] -> [_ _ _ w593 _]
                tunnel: w458 -> [_ _ _ _ w606]
                tunnel: w457 -> [_ _ _ _ _]
                tunnel: w456 -> [w483 _ _ _ _]
                tunnel: w455 -> [_ _ _ _ w605]
                tunnel: w454 -> [_ _ w557 _ _]
                tunnel: w453 -> [w468 _ _ _ _]
                tunnel: w452 -> [w466 _ _ _ _]
                frame #0 {
                  n242 = local read "Efficiency Standard"() -> (w481:u16)
                  n243 = local read "Load selection"() -> (w487:bool[])
                  n244 = property on="Efficiency Standard" class="Ring (strict)"() -> ("Strings []"=w482:string[])  [unwired: 2 in, 2 out]
                  n245 = Number To Fractional String(number=w466, precision (6)=i16 5) -> (F-format string=w465:cluster{"Stator":string[], "Rotor":string[]})  [unwired: 2 in]
                  n246 = global write "ABB global.vi" "Pass Fail Entries"(w483) -> ()
                  n247 = Number To Fractional String(number=w468, precision (6)=i16 1) -> (F-format string=w472:string)  [unwired: 2 in]
                  n248 = Unbundle By Name(w465) -> ("Stator"=w464:string[], "Rotor"=w460:string[])
                  n249 = Index Array(array=w482, index=w481) -> (element=w474:string)
                  n250 = for {
                    tunnel: w464 -> [w501] mode=indexing
                    tunnel: "PE-S" -> [w498]
                    tunnel: [w495] -> w462 mode=indexing
                    i -> [w500]
                    n251 = Increment(x=w500) -> (x+1=w499:i32)
                    n252 = Number To Decimal String(number=w499) -> (decimal integer string=w497:string)  [unwired: 1 in]
                    n253 = Concatenate Strings(w498, w497) -> (w496:string)
                    n254 = Build Array(w501, w496) -> (w495:string[])
                  }
                  n255 = Boolean To (0,1)(Boolean=w487) -> (0, 1=w486:i16[])
                  n256 = Number To Decimal String(number=w486) -> (decimal integer string=w485:string[])  [unwired: 1 in]
                  n257 = Number To Decimal String(number=w481) -> (decimal integer string=w475:string)  [unwired: 1 in]
                  n258 = for {
                    tunnel: w485 -> [w503] mode=indexing
                    tunnel: [w502] -> w484 mode=indexing
                    i -> [w508]
                    n259 = Increment(x=w508) -> (x+1=w507:i32)
                    n260 = Number To Decimal String(number=w507) -> (decimal integer string=w505:string)  [unwired: 1 in]
                    n261 = Concatenate Strings("PE-B", w505) -> (w504:string)
                    n262 = Build Array(w503, w504) -> (w502:string[])
                  }
                  n263 = Build Array(w472, "PE-ET" ("element")) -> (w470:string[])
                  n264 = Concatenate Strings(w474, ":" ("string"), w475) -> (w479:string)
                  n265 = Build Array(w479, "PE-AA") -> (w476:string[])
                  n266 = for {
                    tunnel: w460 -> [w494] mode=indexing
                    tunnel: "PE-O" -> [w491]
                    tunnel: [w488] -> w459 mode=indexing
                    i -> [w493]
                    n267 = Increment(x=w493) -> (x+1=w492:i32)
                    n268 = Number To Decimal String(number=w492) -> (decimal integer string=w490:string)  [unwired: 1 in]
                    n269 = Concatenate Strings(w491, w490) -> (w489:string)
                    n270 = Build Array(w494, w489) -> (w488:string[])
                  }
                  n271 = global write "ABB global.vi" "PF Remarks"("Remarks") -> ()
                  n272 = Build Array (concatenate)(w476, w484, w470, w462, w459) -> (w477:string[][])
                }
                frame #1 {
                  n273 = local read "Selected Loads (% Rated)"() -> (w521:dbl[])
                  n274 = local read "Efficiency Readings"() -> (w520:dbl[][])
                  n275 = Number To Fractional String(number="Frequency (Hz)", precision (6)=i16 1) -> (F-format string=w512:string)  [unwired: 2 in]
                  n276 = Build Array(w512, "PE-F1") -> (w511:string[])
                  n277 = for {
                    tunnel: w521 -> [w541] mode=indexing
                    tunnel: [w543] -> w518 mode=indexing
                    i -> [w546]
                    n278 = Increment(x=w546) -> (x+1=w545:i32)
                    n279 = Number To Decimal String(number=w545) -> (decimal integer string=w538:string)  [unwired: 1 in]
                    n280 = Number To Fractional String(number=w541, precision (6)=i16 1) -> (F-format string=w539:string)  [unwired: 2 in]
                    n281 = Concatenate Strings("PE-L", w538) -> (w540:string)
                    n282 = Build Array(w539, w540) -> (w543:string[])
                  }
                  n283 = Build Array (concatenate)(w516, w518) -> (w517:string[][])
                  n284 = Build Array (concatenate)(w517, w511) -> (w509:string[][])
                  n285 = for {
                    tunnel: w520 -> [w526] mode=indexing
                    tunnel: string[] ["PE-Z", "PE-M", "PE-I", "PE-C", "PE-R", "PE-Y", "PE-T", "PE-W", "PE-J"] -> [w525] mode=indexing
                    shift-right: [w523] -> w510
                    shift-left: w509 -> [w524]
                    n286 = for {
                      tunnel: w526 -> [w529] mode=indexing
                      tunnel: w525 -> [w534]
                      tunnel: [w533] -> w522 mode=indexing
                      i -> [w535]
                      n287 = Increment(x=w535) -> (x+1=w536:i32)
                      n288 = Build Array(w529) -> (w528:dbl[])
                      n289 = Number To Decimal String(number=w536) -> (decimal integer string=w537:string)  [unwired: 1 in]
                      n290 = call "ABB #s to strings.vi"("# type"=enum16{"Float", "Relative time HH:MM"}."Float", "Precision"=i16 4 ("precision (6)"), "Numbers in"=w528) -> ("Strings out"=w531:string[])  [unwired: 8 in]
                      n291 = Concatenate Strings(w534, w537) -> (w532:string)
                      n292 = Build Array (concatenate)(w531, w532) -> (w533:string[])
                    }
                    n293 = Build Array (concatenate)(w524, w522) -> (w523:string[][])
                  }
                }
                frame #2 {
                  n294 = local read "Load selection"() -> (w558:bool[])
                  n295 = Unbundle By Name(w557) -> ("Mech Loss"=w556:dbl, "Total No load Power"=w555:dbl, "No-Load Current"=w554:dbl, "Iron loss"=w553:dbl)
                  n296 = global write "ABB global.vi" "Effy Load Selection"(w558) -> ()
                  n297 = local read "Specified Efficiencies (%)"() -> (w560:dbl[])
                  n298 = local read "Specified  Power Factor"() -> (w565:dbl[])
                  n299 = Build Array(w556, w555, w554, w553) -> (w551:dbl[])
                  n300 = for {
                    tunnel: w560 -> [w573] mode=indexing
                    tunnel: "PE-E" -> [w574]
                    tunnel: [w571] -> w559 mode=indexing
                    i -> [w575]
                    n301 = Increment(x=w575) -> (x+1=w576:i32)
                    n302 = Number To Decimal String(number=w576) -> (decimal integer string=w577:string)  [unwired: 1 in]
                    n303 = Number To Fractional String(number=w573, precision (6)=i16 4) -> (F-format string=w570:string)  [unwired: 2 in]
                    n304 = Concatenate Strings(w574, w577) -> (w569:string)
                    n305 = Build Array(w570, w569) -> (w571:string[])
                  }
                  n306 = Number To Fractional String(number=w551, precision (6)=i16 1) -> (F-format string=w549:string[])  [unwired: 2 in]
                  n307 = for {
                    tunnel: string[] ["PE-NM", "PE-NW", "PE-NA", "PE-NF"] -> [w567] mode=indexing
                    tunnel: w549 -> [w568] mode=indexing
                    tunnel: [w566] -> w548 mode=indexing
                    n308 = Build Array(w568, w567) -> (w566:string[])
                  }
                  n309 = for {
                    tunnel: w565 -> [w582] mode=indexing
                    tunnel: "PE-P" -> [w583]
                    tunnel: [w580] -> w562 mode=indexing
                    i -> [w584]
                    n310 = Increment(x=w584) -> (x+1=w585:i32)
                    n311 = Number To Decimal String(number=w585) -> (decimal integer string=w586:string)  [unwired: 1 in]
                    n312 = Number To Fractional String(number=w582, precision (6)=i16 4) -> (F-format string=w579:string)  [unwired: 2 in]
                    n313 = Concatenate Strings(w583, w586) -> (w578:string)
                    n314 = Build Array(w579, w578) -> (w580:string[])
                  }
                  n315 = Build Array (concatenate)(w559, w563, w562, w548) -> (w547:string[][])
                }
                frame #3 {
                  n316 = local read "Slip Source"() -> (w588:enum16{"Calculated", "Entered"})
                  n317 = local read "Slip Entry"() -> (w595:dbl[])
                  n318 = for {
                    tunnel: w595 -> [w600] mode=indexing
                    tunnel: "PE-Q" -> [w601]
                    tunnel: [w598] -> w592 mode=indexing
                    i -> [w602]
                    n319 = Increment(x=w602) -> (x+1=w603:i32)
                    n320 = Number To Decimal String(number=w603) -> (decimal integer string=w604:string)  [unwired: 1 in]
                    n321 = Number To Fractional String(number=w600, precision (6)=i16 4) -> (F-format string=w597:string)  [unwired: 2 in]
                    n322 = Concatenate Strings(w601, w604) -> (w596:string)
                    n323 = Build Array(w597, w596) -> (w598:string[])
                  }
                  n324 = Number To Decimal String(number=w588) -> (decimal integer string=w589:string)  [unwired: 1 in]
                  n325 = Build Array(w589, "PE-XN") -> (w587:string[])
                  n326 = Build Array (concatenate)(w593, w587, w592) -> (w591:string[][])
                  n327 = global write "ABB global.vi" "Effiy entries"(w591) -> ()
                }
                frame #4 {
                  n328 = case shown="False" w605 {
                    tunnel: w606 -> [w608 _]
                    frame False {
                      n329 = call "ABB Load-Save results.vi"("Path"=w608, "Mode"=enum16{"LOAD", "Save"}."Save") -> ()  [unwired: 10 in]
                    }
                    frame True {
                    }
                  }
                }
              }
            }
          }
        }
        frame True {
        }
      }
    }
  }
